vi "Get Owner.vi"(11 "Game in":refnum<class "Game.lvclass">) -> (2 "Owner":refnum<class "Entity.lvclass">)   [LabVIEW 2020, in "Conditum-Example.lvlib" / "Game.lvclass"]
uses:
  Game.lvclass
  Conditum/Columns/Entity/Entity C.lvclass
  Conditum/Entity/Entity.lvclass
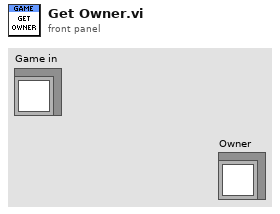
[diagram p1: front panel]
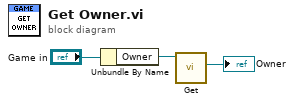
[diagram p0: block diagram]
diagram:
  n1 = Unbundle By Name("Game in") -> ("Owner"=w2:refnum<class "Entity C.lvclass">)
  n2 = call "Get.vi"("Entity in"=w2) -> ("Value"=→"Owner":refnum<class "Entity.lvclass">)  [unwired: 10 in]
